vi "r2.vi"   [LabVIEW 2019]
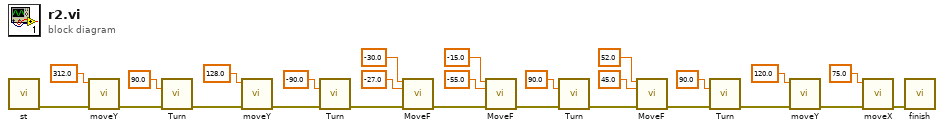
[diagram p0: block diagram]
diagram:
  n1 = call "st.vi"() -> ("Error/Flow Out"=w26:errorcluster)  [unwired: 11 in]
  n2 = call "moveY.vi"("error in (no error)"=w26, "Y"=312.0) -> ("error out"=w24:errorcluster)  [unwired: 9 in]
  n3 = call "Turn.vi"("¨¤«×"=90.0, "error in (no error)"=w24) -> ("error out"=w21:errorcluster)  [unwired: 13 in]
  n4 = call "moveY.vi"("error in (no error)"=w21, "Y"=128.0) -> ("error out"=w19:errorcluster)  [unwired: 9 in]
  n5 = call "Turn.vi"("¨¤«×"=-90.0, "error in (no error)"=w19) -> ("error out"=w18:errorcluster)  [unwired: 13 in]
  n6 = call "MoveF.vi"("X"=-30.0, "Y"=-27.0, "error in (no error)"=w18) -> ("error out"=w13:errorcluster)  [unwired: 12 in]
  n7 = call "MoveF.vi"("X"=-15.0, "Y"=-55.0, "error in (no error)"=w13) -> ("error out"=w11:errorcluster)  [unwired: 12 in]
  n8 = call "Turn.vi"("¨¤«×"=90.0, "error in (no error)"=w11) -> ("error out"=w8:errorcluster)  [unwired: 13 in]
  n9 = call "MoveF.vi"("X"=52.0, "Y"=45.0, "error in (no error)"=w8) -> ("error out"=w6:errorcluster)  [unwired: 12 in]
  n10 = call "Turn.vi"("¨¤«×"=90.0, "error in (no error)"=w6) -> ("error out"=w4:errorcluster)  [unwired: 13 in]
  n11 = call "moveY.vi"("error in (no error)"=w4, "Y"=120.0) -> ("error out"=w3:errorcluster)  [unwired: 9 in]
  n12 = call "moveX.vi"("error in (no error)"=w3, "X"=75.0) -> ("error out"=w2:errorcluster)  [unwired: 9 in]
  n13 = call "finish.vi"("Error/Flow In"=w2) -> ()  [unwired: 11 in]
